vi "Config Type.vi"(11 "LowLimit Condition in":refnum<class "LowLimit Condition.lvclass">) -> (2 "Condition Config":refnum<class "Condition Config.lvclass">)   [LabVIEW 2020, in "VolatusSeq.lvlib" / "LowLimit Condition.lvclass"]
uses:
  LowLimit Condition.lvclass
  LowLimit Condition.lvclass/LowLimit Condition.ctl
  VolatusSeqConfig/LowLimit Condition Config/LowLimit Condition Config.lvclass
  C:/dev/lv20CE/relink/lv-volatus/VolatusSeqConfig/Condition Config/Condition Config.lvclass
  C:/dev/lv20CE/relink/lv-volatus/VolatusSeqConfig/LowLimit Condition Config/LowLimit Condition Config.lvclass
  VolatusSeqConfig/Condition Config/Condition Config.lvclass
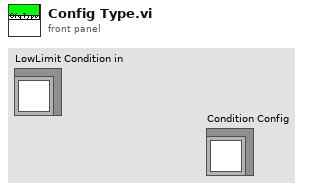
[diagram p1: front panel]
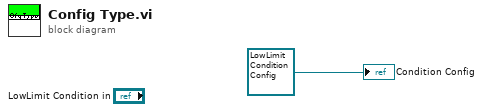
[diagram p0: block diagram]
diagram:
  "Condition Config" <- refnum<class "LowLimit Condition Config.lvclass"> refnum ("VolatusSeqConfig.lvlib:LowLimit Condition Config.lvclass")
